vi "Robot Global Data.vi"() -> ()   [LabVIEW 2015]
doc: "This global VI can contain as many global variables as you need. Place a control on the panel, give it a good name. To read or write to it from a VI, drag the icon to the diagram of that VI. You can also drag from the project. Click on the node to change which global you access. You shouldn't have multiple locations writing to a global or it will cause a race-condition."
uses:
  <vilib>/Rock Robotics/WPI/Camera/WPI_CameraImageSize.ctl
  <vilib>/Rock Robotics/WPI/DriverStation/WPI_DriverStationRobotMode2.ctl
panel:
  in  "WaitTime":dbl
  out "VZ":dbl
  out "VY":dbl
  out "VX":dbl
  in  "JY2 0":bool
  in  "JY1 1":bool
  in  "JY1 0":bool
  out "LinAccZ":dbl
  out "LinAccY":dbl
  out "LinAccX":dbl
  out "Yaw":dbl
  out "Reverse":dbl
  out "JY2 Z":dbl
  out "JY2 Y":dbl
  out "JY2 X":dbl
  out "JY1 Z":dbl
  out "JY1 Y":dbl
  out "JY1 X":dbl
  in  "Robot Mode":T1
  in  "image size":T2=enum."320x240"
  in  "Enable Vision":bool
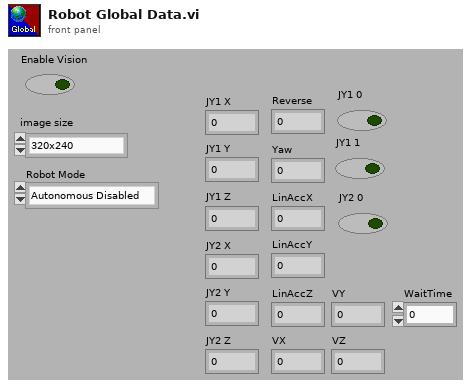
[diagram p1: front panel]
types:
  T1 = typedef "WPI_DriverStationRobotMode2.ctl" = enum16{"Autonomous Disabled", "Autonomous Enabled", "Teleop Disabled", "Teleop Enabled", "Disconnected", "Finish", "Test Disabled", "Test Enabled", "Emergency Stopped"}
  T2 = typedef "WPI_CameraImageSize.ctl" = enum16{"640x480", "320x240", "160x120", "Custom"}
diagram:
